vi "Import Frames.vi"(8 "error in (no error)":errorcluster, 11 "Node Ptr":u64 format="%.0x") -> (0 "error out":errorcluster)   [LabVIEW 2019, in "Diagnostics Addon System Explorer.lvlib"]
uses:
  Diagnostics Addon System Explorer.lvlib
  Types/Frame.Export.ctl
  Shared/Types/Signal.ctl
  Shared/SubVIs/Constants.vi
  <vilib>/NI VeriStand/Custom Device API/NI VeriStand - Get Item Parent.vi
  <vilib>/NI VeriStand/Custom Device API/Custom Device API.lvlib
  Shared/Diagnostics Addon Shared.lvlib
  <vilib>/NI VeriStand/Custom Device Tools/Custom Device Utility Library/Custom Device Utility Library.lvlib
panel:
  in  "Tag":string
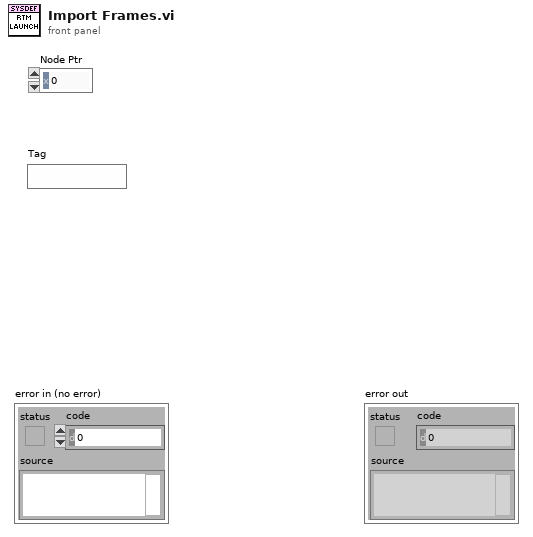
[diagram p1: front panel]
types:
  T1 = typedef "Diagnostics Addon System Explorer.lvlib/Frame.Export.ctl" = cluster{"Name":string, "Description":string, "ID":u32, "Signals":T2[]}
  T2 = typedef "Diagnostics Addon Shared.lvlib/Signal.ctl" = cluster{"Start Bit":u32, "Length":u32, "Scaling Factor":dbl, "Scaling Offset":dbl, "Minimum":dbl, "Maximum":dbl, "Data Type":u32, "Byte Order":u32, "Default Value":dbl, "Name":string, "Units":string, "Description":string}
  T3 = typedef "Custom Device API.lvlib/Custom Device Item Ref.ctl" = u64
  T4 = typedef "Custom Device API.lvlib/Custom Device Item Info.ctl" = cluster{"Name":string, "Is Channel":bool, "GUID":string, "Is Waveform":bool}
  T5 = typedef "Diagnostics Addon Shared.lvlib/Type.ctl" = enum16{"DID", "CDID", "PID", "CPID", "Read Memory", "Write Memory", "DTC Control", "IO Cmd", "IO Resp", "Routine Start Cmd", "Routine Start Resp", "Routine Request Cmd", "Routine Request Resp", "Routine Stop Cmd", "Routine Stop Resp", "UserDefined Cmd", "UserDefined Rsp"}
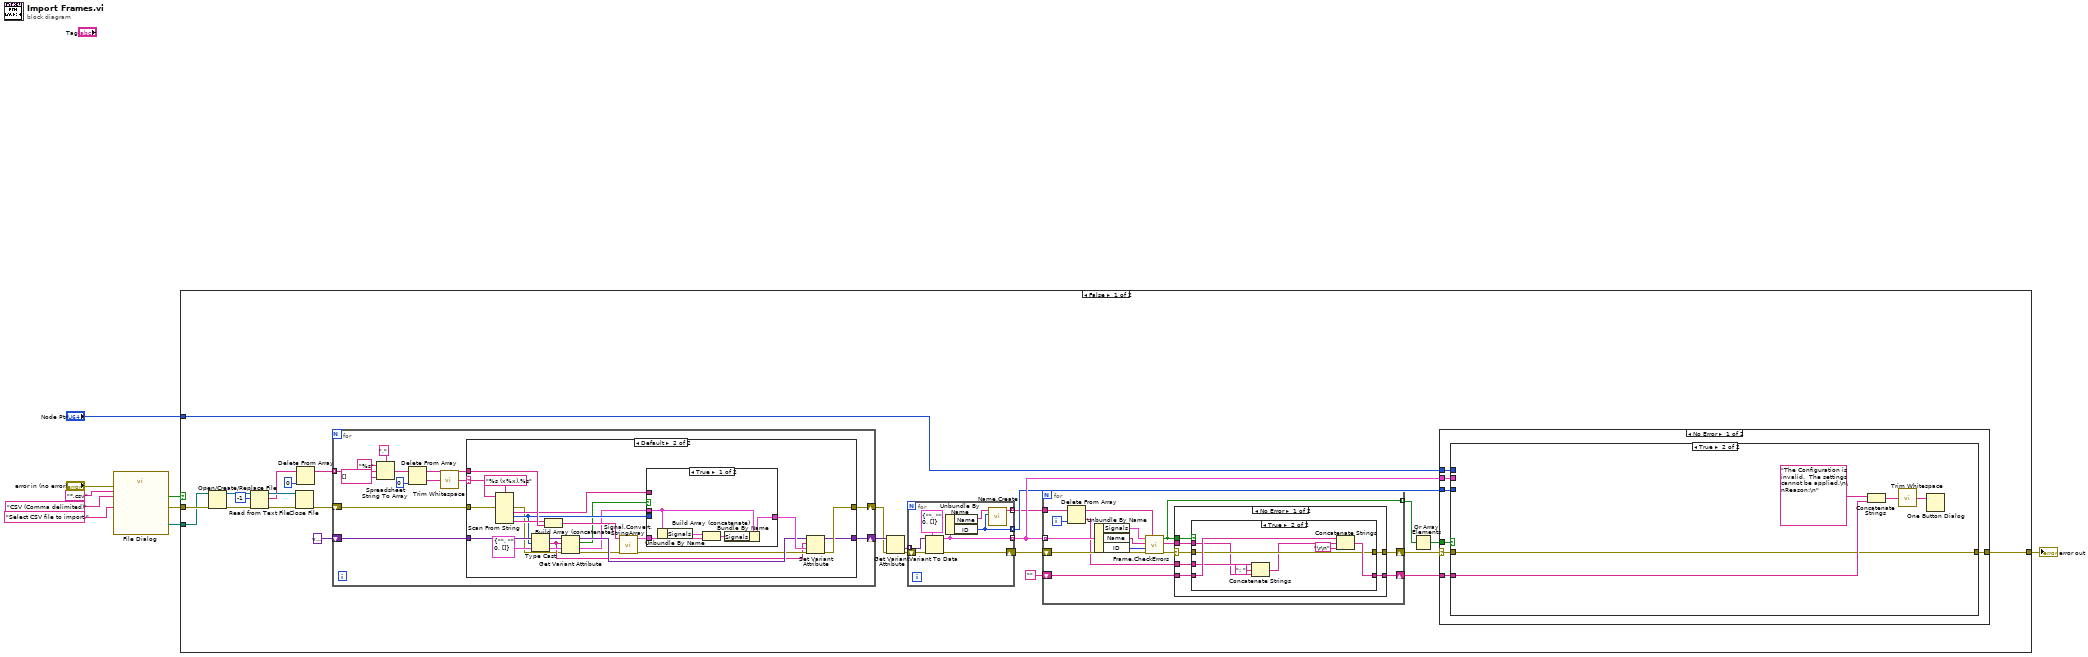
[diagram p0: block diagram]
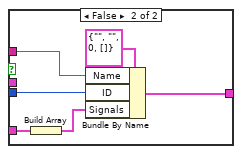
[diagram p3: hidden frame]
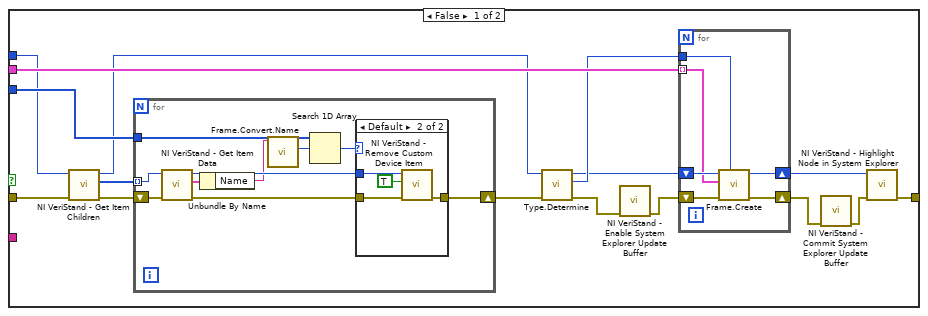
[diagram p4: hidden frame]
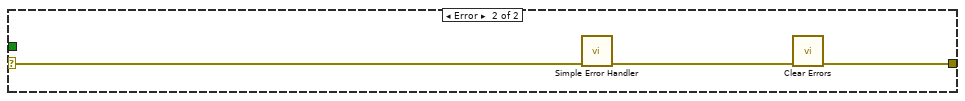
[diagram p6: hidden frame]
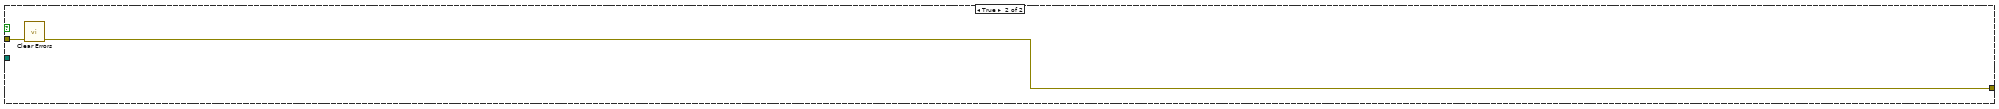
[diagram p9: hidden frame]
diagram:
  n1 = call "File Dialog"("prompt"="Select CSV file to import.", "error in"="error in (no error)", "pattern (all files)"="*.csv" ("pattern label"), "pattern label"="CSV (Comma delimited)") -> ("selected path"=w4:path, "cancelled"=w6:bool, "error out"=w5:errorcluster)  [unwired: 8 in, 1 out]
  n2 = case shown="False" w6 {
    tunnel: w5 -> [w32 w179]
    tunnel: w4 -> [w31 _]
    tunnel: "Node Ptr" -> [w14 _]
    tunnel: [w16 w178] -> w2
    frame False {
      n3 = Open/Create/Replace File(file path (use dialog)=w31, error in=w32) -> (refnum out=w35:refnum<file>, error out=w36:errorcluster)  [unwired: 4 in, 1 out]
      n4 = Read from Text File(file (use dialog)=w35, count=-1, error in=w36) -> (refnum out=w34:refnum<file>, text=w23:string[], error out=w33:errorcluster)  [unwired: 1 in, 1 out]
      n5 = Close File(refnum=w34, error in=w33) -> (error out=w29:errorcluster)  [unwired: 1 out]
      n6 = Delete From Array(array=w23, index=0) -> (array with subset deleted=w11:string[])  [unwired: 1 in, 1 out]
      n7 = for {
        tunnel: w11 -> [w49] mode=indexing
        shift-right: [w40] -> w26
        shift-left: w29 -> [w41]
        shift-right: [w39] -> w27
        shift-left: variant -> [w42]
        n8 = Spreadsheet String To Array(delimiter (Tab)=",", format string="%s", spreadsheet string=w49, array type (2D Dbl)=string[] []) -> (array=w45:string[])
        n9 = Delete From Array(array=w45, index=0) -> (deleted portion=w38:string, array with subset deleted=w44:string[])  [unwired: 1 in]
        n10 = call <vilib>:"Trim Whitespace.vi"("string"=w38) -> ("trimmed string"=w37:string)  [unwired: 1 in]
        n11 = case shown="Default" w37 {
          selector: w37 -> [_ w52]
          tunnel: w44 -> [_ w72]
          tunnel: w42 -> [w51 w66]
          tunnel: w41 -> [w50 w65]
          tunnel: [w50 w59] -> w40
          tunnel: [w51 w58] -> w39
          frame "" {
          }
          frame Default {
            n12 = Scan From String(format string="%s (x%x).%s", input string=w52, error in=w65) -> (error out=w56:errorcluster, output 1=w69:string, output 2=w63:u32, output 3=w67:string)  [unwired: 4 in, 2 out]
            n13 = Type Cast(x=w63) -> (*(type *) &x=w57:string)  [unwired: 1 in]
            n14 = Build Array (concatenate)(w67, w72) -> (w68:string[])
            n15 = Get Variant Attribute(Variant=w66, name=w57, default value (empty Variant)=T1 {"Name"="", "Description"="", "ID"=0, "Signals"=[]} ("DIDPID"), error in=w56) -> (duplicate Variant=w61:variant, found=w54:bool, value=w53:T1, error out=w55:errorcluster)
            n16 = call "Signal.Convert.StringArray.vi"("error in (no error)"=w55, "Signal Parameters"=w68) -> ("error out"=w60:errorcluster, "Signal Parameters"=w70:T2)  [unwired: 8 in]
            n17 = case shown="True" w54 {
              tunnel: w70 -> [w75 w82]
              tunnel: w69 -> [_ w81]
              tunnel: w63 -> [_ w79]
              tunnel: [w73 w78] -> w62
              tunnel: w53 -> [w77 _]
              frame True {
                n18 = Unbundle By Name(w77) -> ("Signals"=w76:T2[])
                n19 = Build Array (concatenate)(w76, w75) -> (w74:T2[])
                n20 = Bundle By Name(cluster=w77, "Signals"=w74) -> (w73:T1)
              }
              frame False {
                n21 = Build Array(w82) -> (w80:T2[])
                n22 = Bundle By Name(cluster=T1 {"Name"="", "Description"="", "ID"=0, "Signals"=[]} ("DIDPID"), "Name"=w81, "ID"=w79, "Signals"=w80) -> (w78:T1)
              }
            }
            n23 = Set Variant Attribute(Variant=w61, name=w57, value=w62, error in=w60) -> (Variant out=w58:variant, error out=w59:errorcluster)  [unwired: 1 out]
          }
        }
      }
      n24 = Get Variant Attribute(Variant=w27, error in=w26) -> (values=w25:variant[], error out=w24:errorcluster)  [unwired: 2 in, 2 out]
      n25 = for {
        tunnel: w25 -> [w90] mode=indexing
        shift-right: [w88] -> w15
        shift-left: w24 -> [w89]
        tunnel: [w87] -> w17 mode=indexing
        tunnel: [w86] -> w13 mode=indexing
        tunnel: [w84] -> w10 mode=indexing
        n26 = Variant To Data(error in=w89, type=T1 {"Name"="", "Description"="", "ID"=0, "Signals"=[]} ("DIDPID"), Variant=w90) -> (data=w87:T1, error out=w88:errorcluster)
        n27 = Unbundle By Name(w87) -> ("Name"=w85:string, "ID"=w86:u32)
        n28 = call "Name.Create.vi"("PID Number"=w86, "PID Name"=w85) -> ("VS Name"=w84:string)  [unwired: 9 in]
      }
      n29 = for {
        tunnel: w17 -> [w158] mode=indexing
        shift-right: [w149] -> w12
        shift-left: w15 -> [w154]
        shift-right: [w152] -> w18
        shift-left: "" -> [w151]
        tunnel: [w148] -> w20 mode=indexing
        tunnel: w10 -> [w147]
        i -> [w146]
        n30 = Delete From Array(array=w147, index=w146) -> (deleted portion=w144:string, array with subset deleted=w145:string[])  [unwired: 1 in]
        n31 = Unbundle By Name(w158) -> ("Signals"=w155:T2[], "Name"=w157:string, "ID"=w156:u32)
        n32 = call "Frame.CheckErrors.vi"("Existing PIDs"=w145, "error in (no error)"=w154, "ID"=w156, "Name"=w157, "Signals"=w155) -> ("error out"=w150:errorcluster, "Error Type"=w153:string, "Error?"=w148:bool)  [unwired: 4 in]
        n33 = case shown="No Error" w150 {
          selector: w150 -> [w161 w176]
          tunnel: w148 -> [w164 _]
          tunnel: w153 -> [w165 _]
          tunnel: [w163 w177] -> w152
          tunnel: w151 -> [w162 w177]
          tunnel: [w160 w176] -> w149
          tunnel: w144 -> [w159 _]
          frame No Error {
            n34 = case shown="True" w164 {
              tunnel: w165 -> [_ w169]
              tunnel: [w167 w175] -> w163
              tunnel: w162 -> [w167 w174]
              tunnel: w161 -> [w166 w172]
              tunnel: [w166 w172] -> w160
              tunnel: w159 -> [_ w171]
              frame False {
              }
              frame True {
                n35 = Concatenate Strings(w171, ": " ("string"), w169) -> (w168:string)
                n36 = Concatenate Strings(w174, w168, "\r\n") -> (w175:string)
              }
            }
          }
          frame Error {
          }
        }
      }
      n37 = Or Array Elements(Boolean array=w20) -> (logical OR=w19:bool)
      n38 = case shown="No Error" w12 {
        selector: w12 -> [w94 w143]
        tunnel: w19 -> [w98 _]
        tunnel: w18 -> [w97 _]
        tunnel: w17 -> [w96 _]
        tunnel: [w95 w141] -> w16
        tunnel: w14 -> [w93 _]
        tunnel: w13 -> [w92 _]
        frame No Error {
          n39 = case shown="True" w98 {
            tunnel: w97 -> [_ w138]
            tunnel: w94 -> [w104 w137]
            tunnel: w96 -> [w110 _]
            tunnel: [w109 w137] -> w95
            tunnel: w93 -> [w101 _]
            tunnel: w92 -> [w105 _]
            frame False {
              n40 = call <vilib>:"NI VeriStand - Get Item Children.vi"("error in (no error)"=w104, "Item Ref in"=w101) -> ("error out"=w107:errorcluster, "Child Refs"=w106:T3[], "Item Ref out"=w100:T3)  [unwired: 6 in, 1 out]
              n41 = for {
                shift-right: [w119] -> w103
                shift-left: w107 -> [w123]
                tunnel: w106 -> [w122] mode=indexing
                tunnel: w105 -> [w121]
                n42 = call <vilib>:"NI VeriStand - Get Item Data.vi"("error in (no error)"=w123, "Item Ref in"=w122) -> ("error out"=w120:errorcluster, "Item Info"=w124:T4, "Item Ref out"=w118:T3)  [unwired: 7 out]
                n43 = Unbundle By Name(w124) -> ("Name"=w116:string)
                n44 = call "Frame.Convert.Name.vi"("VS Frame Name"=w116) -> ("ID"=w115:u16)  [unwired: 9 in, 1 out]
                n45 = Search 1D Array(1D array=w121, element=w115) -> (index of element=w117:i32)  [unwired: 1 in]
                n46 = case shown="Default" w117 {
                  tunnel: w120 -> [w125 w129]
                  tunnel: [w125 w128] -> w119
                  tunnel: w118 -> [_ w127]
                  frame -1 {
                  }
                  frame Default {
                    n47 = call <vilib>:"NI VeriStand - Remove Custom Device Item.vi"("error in (no error)"=w129, "Force Delete (F)"=TRUE, "Item Ref in"=w127) -> ("error out"=w128:errorcluster)  [unwired: 7 in, 1 out]
                  }
                }
              }
              n48 = call "Type.Determine.vi"("error in (no error)"=w103, "Node Ptr"=w100) -> ("error out"=w102:errorcluster, "Type"=w108:T5, "Item Ref out"=w99:T3)  [unwired: 6 in, 1 out]
              n49 = call <vilib>:"NI VeriStand - Enable System Explorer Update Buffer.vi"("error in (no error)"=w102) -> ("error out"=w113:errorcluster)  [unwired: 10 in]
              n50 = for {
                tunnel: w108 -> [w132]
                shift-right: [w133] -> w112
                shift-left: w113 -> [w134]
                shift-right: [w135] -> w114
                shift-left: w99 -> [w131]
                tunnel: w110 -> [w130] mode=indexing
                n51 = call "Frame.Create.vi"("Type"=w132, "error in (no error)"=w134, "Frame"=w130, "Section Ptr"=w131) -> ("error out"=w133:errorcluster, "Parent Ref out"=w135:T3)  [unwired: 6 in]
              }
              n52 = call <vilib>:"NI VeriStand - Commit System Explorer Update Buffer.vi"("error in (no error)"=w112) -> ("error out"=w111:errorcluster)  [unwired: 10 in]
              n53 = call <vilib>:"NI VeriStand - Highlight Node in System Explorer.vi"("error in (no error)"=w111, "Item Ref in"=w114) -> ("error out"=w109:errorcluster)  [unwired: 8 in, 1 out]
            }
            frame True {
              n54 = Concatenate Strings("The Configuration is invalid.  The settings cannot be applied.\n\nReason:\n" ("message"), w138) -> (w140:string)
              n55 = call <vilib>:"Trim Whitespace.vi"("string"=w140) -> ("trimmed string"=w136:string)  [unwired: 1 in]
              n56 = One Button Dialog(message=w136) -> ()  [unwired: 1 in, 1 out]
            }
          }
        }
        frame Error {
          n57 = call <vilib>:"Simple Error Handler.vi"("error in (no error)"=w143) -> ("error out"=w142:errorcluster)  [unwired: 4 in, 4 out]
          n58 = call <vilib>:"Clear Errors.vi"("error in (no error)"=w142) -> ("error out"=w141:errorcluster)  [unwired: 5 in, 1 out]
        }
      }
    }
    frame True {
      n59 = call <vilib>:"Clear Errors.vi"("error in (no error)"=w179) -> ("error out"=w178:errorcluster)  [unwired: 5 in, 1 out]
    }
  }
  "error out" <- w2
